vi "Programacion 8 Lester Roche.vi"() -> ()   [LabVIEW 2011]
panel:
  out "Contador":dbl
  out "Temper 36-60":dbl
  out "Temper 21-35":dbl
  out "Temper 1-20":dbl
  out "Temperatura":i32(slide) scale=0.0..60.0
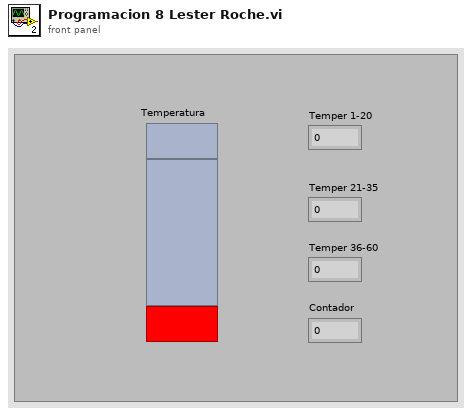
[diagram p1: front panel]
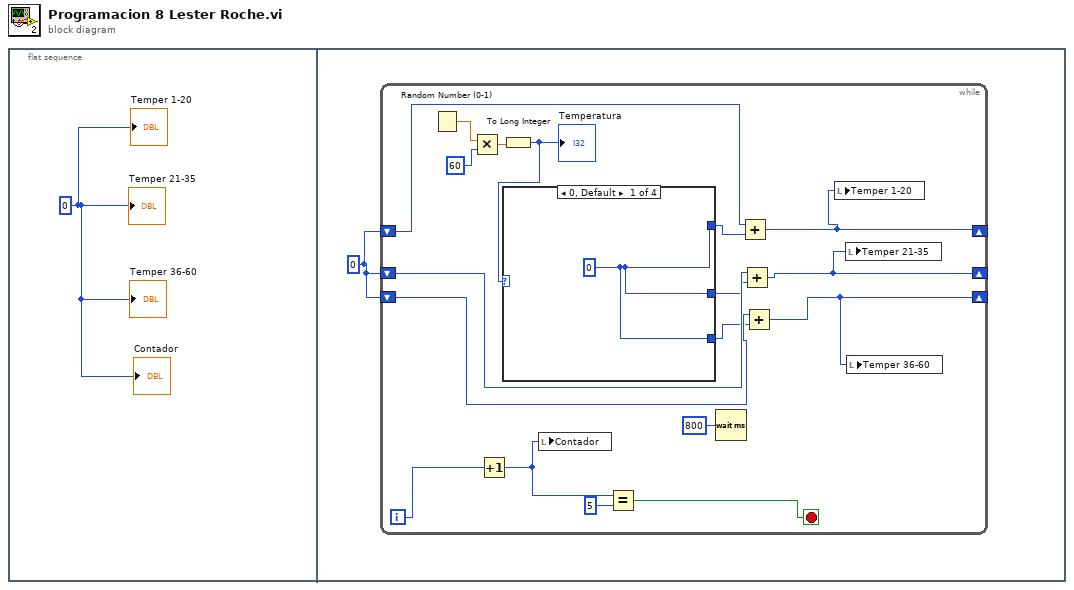
[diagram p0: block diagram]
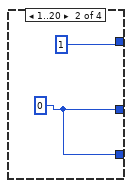
[diagram p2: hidden frame]
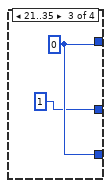
[diagram p3: hidden frame]
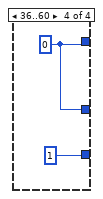
[diagram p4: hidden frame]
diagram:
  n1 = flat-sequence {
    frame #0 {
      w1 = 0
      "Temper 1-20" <- w1
      "Temper 21-35" <- w1
      "Temper 36-60" <- w1
      "Contador" <- w1
    }
    frame #1 {
      w2 = 0
      n2 = while {
        shift-right: [w5] -> _
        shift-left: w2 -> [w11]
        shift-right: [w4] -> _
        shift-left: w2 -> [w9]
        shift-right: [w3] -> _
        shift-left: w2 -> [w7]
        i -> [w18]
        stop <- w15 stop-if-true
        n3 = Random Number (0-1)() -> (number: 0 to 1=w20:dbl)
        n4 = Multiply(x=w20, y=60) -> (x*y=w13:dbl)
        n5 = Increment(x=w18) -> (x+1=w17:i32)
        n6 = To Long Integer(number=w13) -> (32bit integer=w12:i32)
        "Temperatura" <- w12
        n7 = case shown="0, Default" w12 {
          tunnel: [w21 1 w25 w26] -> w10
          tunnel: [w21 w23 1 w26] -> w8
          tunnel: [w21 w23 w25 1] -> w6
          frame 0, Default {
            w21 = 0
          }
          frame 1..20 {
            w23 = 0
          }
          frame 21..35 {
            w25 = 0
          }
          frame 36..60 {
            w26 = 0
          }
        }
        n8 = local write "Contador"(w17) -> ()
        n9 = Equal?(x=w17, y=5) -> (x = y?=w15:bool)
        n10 = Wait (ms)(milliseconds to wait=u32 800) -> ()  [unwired: 1 out]
        n11 = Add(x=w11, y=w10) -> (x+y=w5:i32)
        n12 = Add(x=w9, y=w8) -> (x+y=w4:i32)
        n13 = Add(x=w7, y=w6) -> (x+y=w3:i32)
        n14 = local write "Temper 1-20"(w5) -> ()
        n15 = local write "Temper 21-35"(w4) -> ()
        n16 = local write "Temper 36-60"(w3) -> ()
      }
    }
  }
